vi "ReadWriteTxt.vi"(0 "File Path":path, 5 "InputString":string, 11 "error in (no error)":errorcluster, 13 "FileOperation":T1) -> (4 "StringOut":string, 15 "error out":errorcluster)   [LabVIEW 2021, in "CustomSortPath.lvlib"]
doc: "This Vi gets the file path,input string and file operation as input. It reads or writes a data into a test file."
uses:
  CustomSortPath.lvlib
  Controls/FileOperation.ctl
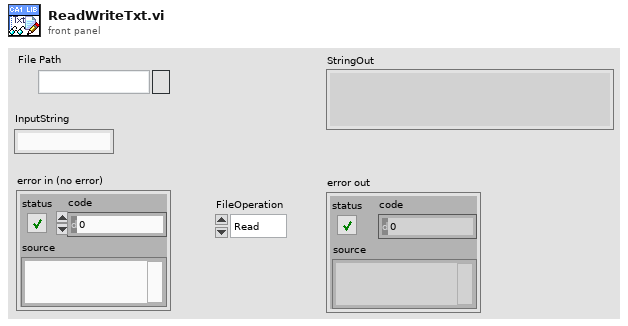
[diagram p1: front panel]
types:
  T1 = typedef "CustomSortPath.lvlib/FileOperation.ctl" = enum16{"Read", "Write"}
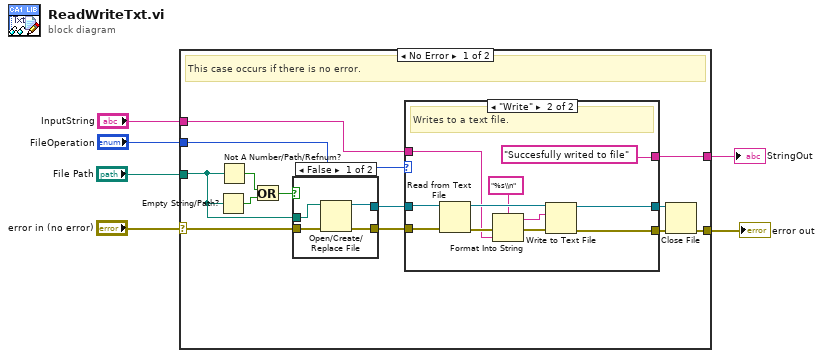
[diagram p0: block diagram]
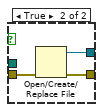
[diagram p2: hidden frame]
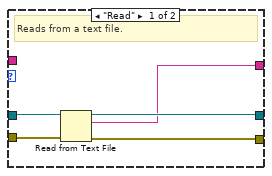
[diagram p3: hidden frame]
diagram:
  n1 = case shown="No Error" "error in (no error)" {
    selector: "error in (no error)" -> [w11 w43]
    tunnel: "File Path" -> [w7 _]
    tunnel: "FileOperation" -> [w19 _]
    tunnel: "InputString" -> [w18 _]
    tunnel: [w17 w43] -> w3
    tunnel: [w16 _] -> w2
    frame No Error {
      # "This case occurs if there is no error."
      n2 = Empty String/Path?(string/path=w7) -> (empty?=w10:bool)
      n3 = Not A Number/Path/Refnum?(number/path/refnum=w7) -> (NaN/Path/Refnum?=w9:bool)
      n4 = Or(x=w9, y=w10) -> (x .or. y?=w8:bool)
      n5 = case shown="False" w8 {
        tunnel: [w22 w26] -> w15
        tunnel: [w21 w25] -> w14
        tunnel: w11 -> [w23 w24]
        tunnel: w7 -> [w20 _]
        frame False {
          n6 = Open/Create/Replace File(file path (use dialog)=w20, error in=w23) -> (refnum out=w21:refnum<file>, error out=w22:errorcluster)  [unwired: 4 in, 1 out]
        }
        frame True {
          n7 = Open/Create/Replace File(error in=w24) -> (refnum out=w25:refnum<file>, error out=w26:errorcluster)  [unwired: 5 in, 1 out]
        }
      }
      n8 = case shown="\"Write\"" w19 {
        tunnel: w15 -> [w31 w40]
        tunnel: [w30 w42] -> w13
        tunnel: w18 -> [_ w34]
        tunnel: w14 -> [w29 w38]
        tunnel: [w28 w41] -> w12
        tunnel: [w27 "Succesfully writed to file"] -> w16
        frame "Read" {
          # "Reads from a text file."
          n9 = Read from Text File(file (use dialog)=w29, error in=w31) -> (refnum out=w28:refnum<file>, text=w27:string, error out=w30:errorcluster)  [unwired: 2 in, 1 out]
        }
        frame "Write" {
          # "Writes to a text file."
          n10 = Read from Text File(file (use dialog)=w38, error in=w40) -> (refnum out=w37:refnum<file>, error out=w39:errorcluster)  [unwired: 2 in, 2 out]
          n11 = Format Into String(format string="%s\\n", error in=w39, w34) -> (resulting string=w33:string, error out=w36:errorcluster)  [unwired: 1 in]
          n12 = Write to Text File(file (use dialog)=w37, text=w33, error in=w36) -> (refnum out=w41:refnum<file>, error out=w42:errorcluster)  [unwired: 1 in, 1 out]
        }
      }
      n13 = Close File(refnum=w12, error in=w13) -> (error out=w17:errorcluster)  [unwired: 1 out]
    }
    frame Error {
      # "This case occurs if there is any error."
    }
  }
  "error out" <- w3
  "StringOut" <- w2
